vi "main.vi"() -> ()   [LabVIEW 2023]
panel:
  out "price":i32
  in  "flavor":string
  in  "count":i32
  in  "member":bool=TRUE
  in  "theta":dbl format="%#_13g"
  in  "b":dbl format="%#_13g"
  in  "a":dbl format="%#_13g"
  in  "r":dbl format="%#_13g"
  in  "shape":string
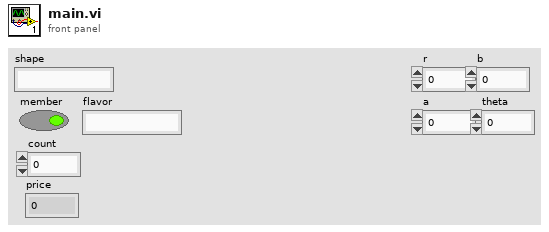
[diagram p1: front panel]
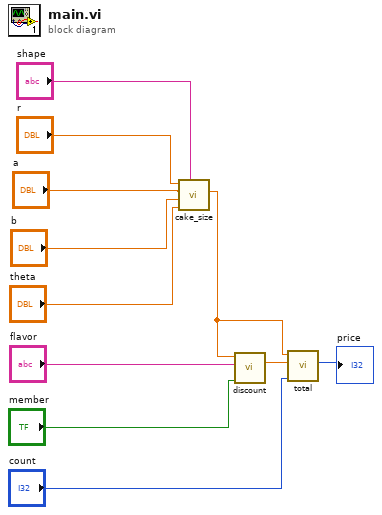
[diagram p0: block diagram]
diagram:
  n1 = call "cake_size.vi"("shape"="shape", "theta"="theta", "b"="b", "a"="a", "r"="r") -> ("size"=w4:dbl)  [unwired: 6 in]
  n2 = call "discount.vi"("member"="member", "flavor"="flavor", "size"=w4) -> ("discount"=w3:dbl)  [unwired: 8 in]
  n3 = call "total.vi"("count"="count", "discount"=w3, "size"=w4) -> ("price"=→"price":i32)  [unwired: 8 in]
